vi "todojunto.vi"() -> ()   [LabVIEW 2018]
uses:
  Control 1.ctl
panel:
  out "contar minusculas":i32
  out "mayuscula ok 2":bool
  out "mayuscula ok":bool
  out "size(s) 2":i32
  out "ERROR":string
  in  "usuario":string
  out "contar mayusculas":i32
  out "contraseña en un vector":u8[](array[numeric])
  in  "OK Button":bool
  in  "CONTRACEÑA":string
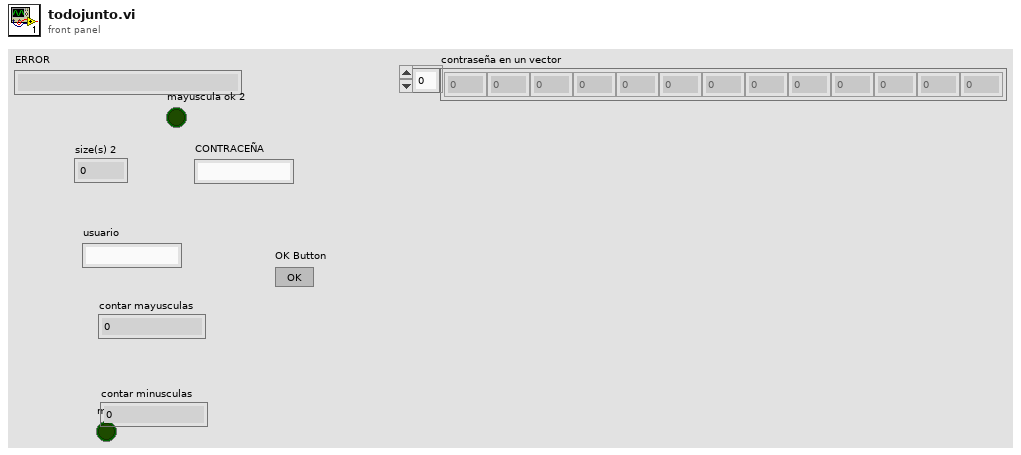
[diagram p1: front panel]
types:
  T1 = typedef "Control 1.ctl" = enum16{"otro", "V. min y MAYU", "control", "V.usuario/contraseña", "V.entre 8 y 16"}
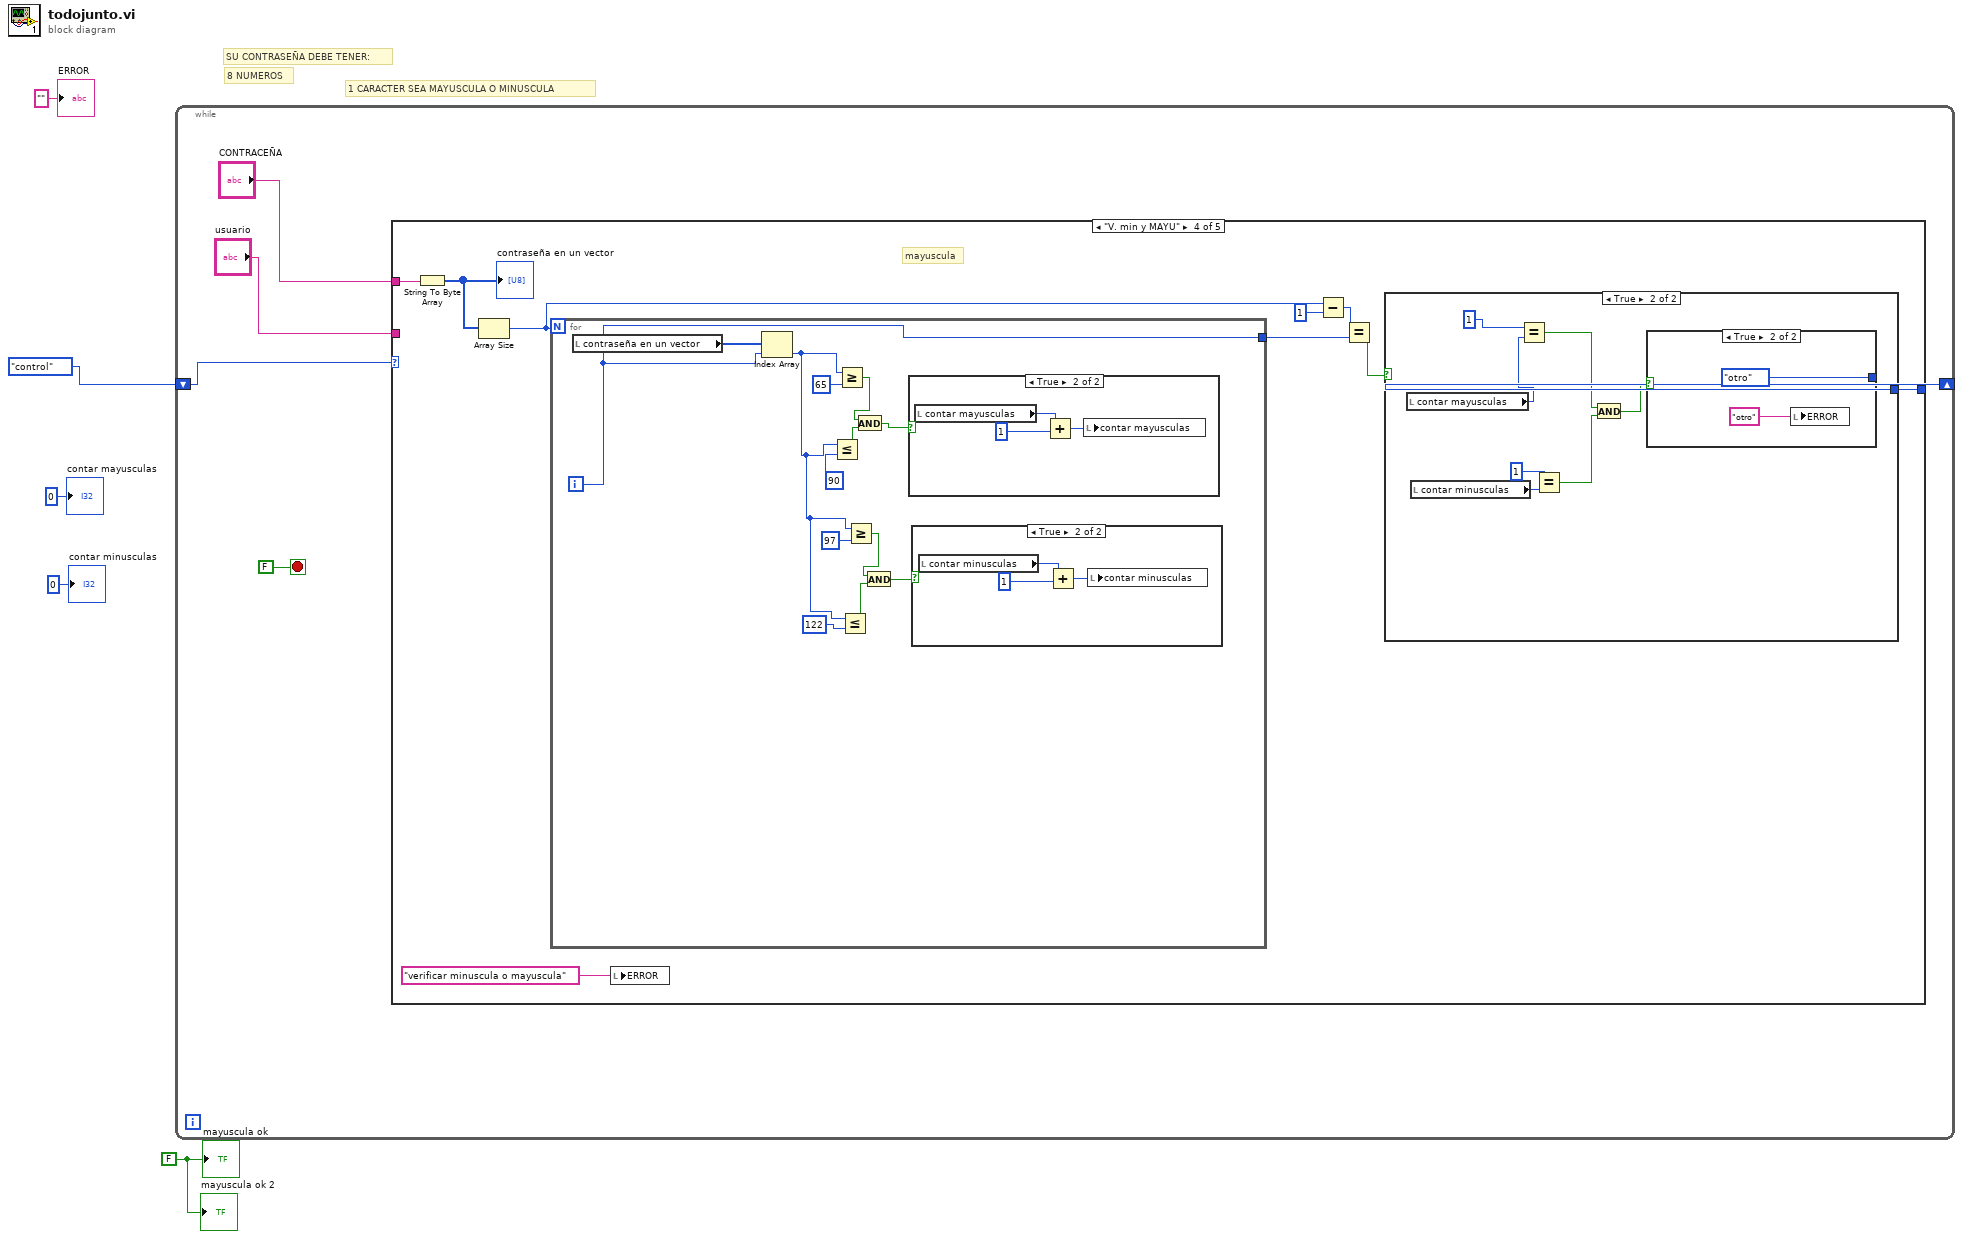
[diagram p0: block diagram]
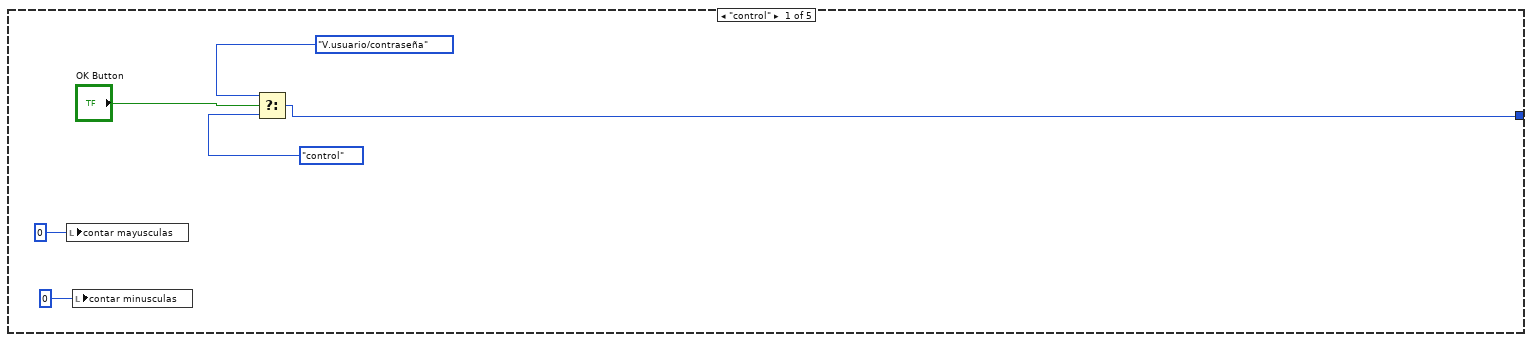
[diagram p2: hidden frame]
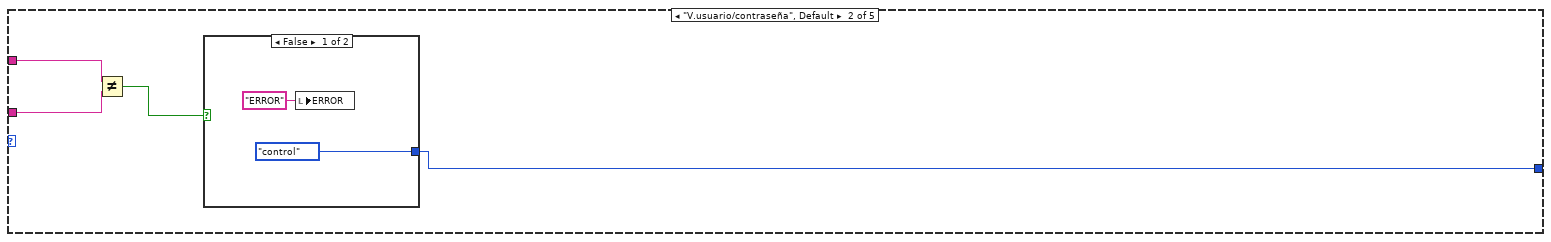
[diagram p3: hidden frame]
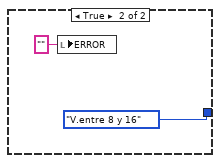
[diagram p4: hidden frame]
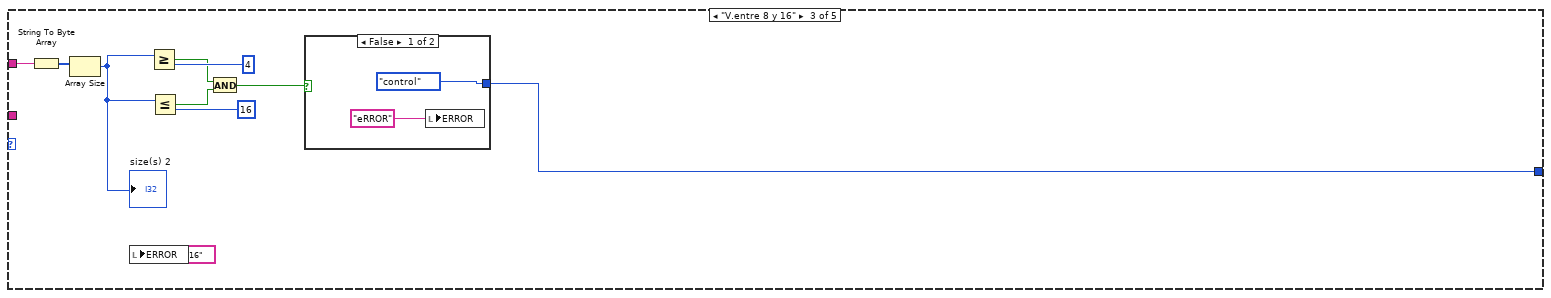
[diagram p5: hidden frame]
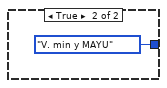
[diagram p6: hidden frame]
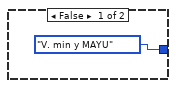
[diagram p7: hidden frame]
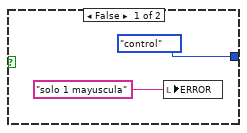
[diagram p8: hidden frame]
diagram:
  w2 = FALSE ("mayuscula ok")
  # "1 CARACTER SEA MAYUSCULA O MINUSCULA"
  # "8 NUMEROS"
  # "SU CONTRASEÑA DEBE TENER:"
  n1 = while {
    shift-right: [w7] -> _
    shift-left: Control_1."control" ("Enum") -> [w9]
    stop <- FALSE stop-if-true
    n2 = case shown="\"V. min y MAYU\"" w9 {
      tunnel: "CONTRACEÑA" -> [_ w20 w33 w45 _]
      tunnel: "usuario" -> [_ w19 _ _ _]
      tunnel: [w16 w17 w25 w39 _] -> w7
      frame "control" {
        n3 = local write "contar mayusculas"(0 ("Numeric")) -> ()
        n4 = local write "contar minusculas"(0 ("Numeric")) -> ()
        n5 = Select(t=Control_1."V.usuario/contraseña" ("Enum"), s="OK Button", f=Control_1."control" ("Enum")) -> (s? t:f=w16:T1)
      }
      frame "V.usuario/contraseña", Default {
        n6 = Not Equal?(x=w20, y=w19) -> (x != y?=w18:bool)
        n7 = case shown="False" w18 {
          tunnel: [Control_1."control" ("Enum") Control_1."V.entre 8 y 16" ("Enum")] -> w17
          frame False {
            n8 = local write "ERROR"("ERROR" ("ERROR")) -> ()
          }
          frame True {
            n9 = local write "ERROR"("" ("ERROR")) -> ()
          }
        }
      }
      frame "V.entre 8 y 16" {
        n10 = String To Byte Array(string=w33) -> (unsigned byte array=w32:u8[])
        n11 = Array Size(array=w32) -> (size(s)=w30:i32)
        "size(s) 2" <- w30
        n12 = local write "ERROR"("verificar 8 o 16" ("ERROR")) -> ()
        n13 = Greater Or Equal?(x=w30, y=4) -> (x >= y?=w28:bool)
        n14 = Less Or Equal?(x=w30, y=16) -> (x <= y?=w27:bool)
        n15 = And(x=w28, y=w27) -> (x .and. y?=w26:bool)
        n16 = case shown="False" w26 {
          tunnel: [Control_1."control" ("Enum") Control_1."V. min y MAYU" ("Enum")] -> w25
          frame False {
            n17 = local write "ERROR"("eRROR" ("ERROR")) -> ()
          }
          frame True {
          }
        }
      }
      frame "V. min y MAYU" {
        # "mayuscula"
        n18 = String To Byte Array(string=w45) -> (unsigned byte array=w44:u8[])
        "contraseña en un vector" <- w44
        n19 = Array Size(array=w44) -> (size(s)=w43:i32)
        n20 = for {
          N: w43 -> [_]
          tunnel: [w61] -> w38
          i -> [w61]
          n21 = local read "contraseña en un vector"() -> (w71:u8[])
          n22 = Index Array(array=w71, index=w61) -> (element=w59:u8)
          n23 = Less Or Equal?(x=w59, y=u8 90 ("lower limit")) -> (x <= y?=w67:bool)
          n24 = Greater Or Equal?(x=w59, y=u8 65 ("upper limit")) -> (x >= y?=w69:bool)
          n25 = Less Or Equal?(x=w59, y=u8 122 ("lower limit")) -> (x <= y?=w65:bool)
          n26 = Greater Or Equal?(x=w59, y=u8 97 ("upper limit")) -> (x >= y?=w63:bool)
          n27 = And(x=w69, y=w67) -> (x .and. y?=w66:bool)
          n28 = And(x=w63, y=w65) -> (x .and. y?=w60:bool)
          n29 = case shown="True" w66 {
            frame False {
            }
            frame True {
              n30 = local read "contar mayusculas"() -> (w77:i32)
              n31 = Add(x=w77, y=1) -> (x+y=w75:i32)
              n32 = local write "contar mayusculas"(w75) -> ()
            }
          }
          n33 = case shown="True" w60 {
            frame False {
            }
            frame True {
              n34 = local read "contar minusculas"() -> (w74:i32)
              n35 = Add(x=w74, y=1) -> (x+y=w72:i32)
              n36 = local write "contar minusculas"(w72) -> ()
            }
          }
        }
        n37 = local write "ERROR"("verificar minuscula o mayuscula" ("ERROR")) -> ()
        n38 = Subtract(x=w43, y=1) -> (x-y=w41:i32)
        n39 = Equal?(x=w41, y=w38) -> (x = y?=w40:bool)
        n40 = case shown="True" w40 {
          tunnel: [Control_1."V. min y MAYU" ("Enum") _] -> w39
          frame False {
          }
          frame True {
            n41 = local read "contar mayusculas"() -> (w53:i32)
            n42 = local read "contar minusculas"() -> (w52:i32)
            n43 = Equal?(x=1 ("y"), y=w53) -> (x = y?=w50:bool)
            n44 = Equal?(x=1, y=w52) -> (x = y?=w49:bool)
            n45 = And(x=w50, y=w49) -> (x .and. y?=w48:bool)
            n46 = case shown="True" w48 {
              tunnel: [Control_1."control" ("Enum") Control_1."otro" ("Enum")] -> _
              frame False {
                n47 = local write "ERROR"("solo 1 mayuscula" ("ERROR")) -> ()
              }
              frame True {
                n48 = local write "ERROR"("otro" ("ERROR")) -> ()
              }
            }
          }
        }
      }
      frame "otro" {
      }
    }
  }
  "contar mayusculas" <- 0 ("Numeric")
  "ERROR" <- "" ("ERROR")
  "mayuscula ok" <- w2
  "mayuscula ok 2" <- w2
  "contar minusculas" <- 0 ("Numeric")
